vi "Data.vi"() -> ()   [LabVIEW 2015]
uses:
  <vilib>/addons/control/pid/pid.llb/PID (DBL).vi
  WINDOWS/system32/wlmData.dll
  <vilib>/addons/control/pid/NI_PID_pid.lvlib
panel:
  in  "output range CH4":cluster{"output high":dbl, "output low":dbl}={"output high"=2.5, "output low"=-2.5}
  in  "output range CH3":cluster{"output high":dbl, "output low":dbl}={"output high"=2.5, "output low"=-2.5}
  in  "output range CH2":cluster{"output high":dbl, "output low":dbl}={"output high"=2.5, "output low"=-2.5}
  in  "output range CH1":cluster{"output high":dbl, "output low":dbl}={"output high"=2.5, "output low"=-2.5}
  in  "Set p2":bool
  in  "Set f CH4 (THz) p2":dbl=811.289308 format="%.6f"
  in  "Set f CH3 (THz) p2":dbl=320.57268 format="%.6f"
  in  "Set f CH2 (THz) p2":dbl=751.527688 format="%.6f"
  in  "Set f CH1 (THz) p2":dbl=405.646266 format="%.6f"
  in  "Set p1":bool
  in  "Set f CH4 (THz) p1":dbl=811.289308 format="%.6f"
  in  "Set f CH3 (THz) p1":dbl=320.56993 format="%.6f"
  in  "Set f CH2 (THz) p1":dbl=751.52853 format="%.6f"
  in  "Set f CH1 (THz) p1":dbl=405.64502 format="%.6f"
  in  "Active interval CH4 (MHz)":dbl=100000.0
  in  "Zero CH4":bool
  in  "PID Out CH4(V)":dbl
  in  "PID gains CH4":T1={"proportional gain (Kc)"=1e-05, "integral time (Ti, min)"=0.0005, "derivative time (Td, min)"=0.0} {"derivative time (Td, min)" format="%.9f"; "integral time (Ti, min)" format="%.9f"; "proportional gain (Kc)" format="%.9f"}
  in  "Reinitialize PID CH4 (F)":bool
  in  "Inverse CH4":bool=TRUE
  out "df CH4 (MHz)":dbl format="%#.1f"
  out "Current f CH4 (THz)":dbl format="%#_9g"
  out "CH4 Reading":bool
  in  "Lock CH4":bool
  in  "Set f CH4 (THz)":dbl=811.289308 format="%.6f"
  out "df CH4 Chart (MHz)":dbl(graph)
  in  "PID Out CH3(V)":dbl
  in  "Zero CH3":bool
  in  "Active interval CH3 (MHz)":dbl=100000.0
  in  "PID gains CH3":T1={"proportional gain (Kc)"=1e-05, "integral time (Ti, min)"=0.0005, "derivative time (Td, min)"=0.0} {"derivative time (Td, min)" format="%.9f"; "integral time (Ti, min)" format="%.9f"; "proportional gain (Kc)" format="%.9f"}
  in  "Reinitialize PID CH3 (F)":bool
  in  "Inverse CH3":bool=TRUE
  out "df CH3 (MHz)":dbl=0.3482338115645689 format="%#.1f"
  out "Current f CH3 (THz)":dbl=320.5699303482334 format="%#_9g"
  out "CH3 Reading":bool
  in  "Lock CH3":bool
  in  "Set f CH3 (THz)":dbl=320.56993 format="%.6f"
  out "df CH3 Chart (MHz)":dbl(graph)=0.3482338115645689
  out "df CH2 Chart (MHz)":dbl(graph)=8543.924245259404
  in  "Zero CH2":bool
  in  "PID Out CH2(V)":dbl min=-10.0 max=10.0
  in  "Zero CH1":bool
  in  "PID Out CH1(V)":dbl
  out "df CH1 Chart (MHz)":dbl(graph)=-366.051154003344
  in  "PID gains CH2":T1={"proportional gain (Kc)"=1e-06, "integral time (Ti, min)"=1e-06, "derivative time (Td, min)"=0.0} {"derivative time (Td, min)" format="%.9f"; "integral time (Ti, min)" format="%.9f"; "proportional gain (Kc)" format="%.9f"}
  in  "Reinitialize PID CH2 (F)":bool
  in  "Inverse CH2":bool=TRUE
  out "df CH2 (MHz)":dbl=8543.924245259404 format="%#.1f"
  out "Current f CH2 (THz)":dbl=751.5362439242452 format="%#_9g"
  out "CH2 Reading":bool
  in  "Lock CH2":bool
  in  "Active interval CH2 (MHz) 2":dbl=100000.0
  in  "Set f CH2 (THz)":dbl=751.52853 format="%.6f"
  in  "Lock CH1":bool
  out "CH1 Reading":bool
  in  "Ch control":string="None"
  in  "Active interval CH1 (MHz)":dbl=100000.0
  out "Current f CH1 (THz)":dbl=405.644653948846 format="%#_9g"
  out "df CH1 (MHz)":dbl=-366.051154003344 format="%#.1f"
  in  "Inverse CH1":bool=TRUE
  in  "Reinitialize PID CH1 (F)":bool
  in  "Set f CH1 (THz)":dbl=405.64502 format="%.6f"
  in  "PID gains CH1":T1={"proportional gain (Kc)"=1e-05, "integral time (Ti, min)"=0.0005, "derivative time (Td, min)"=0.0} {"derivative time (Td, min)" format="%.9f"; "integral time (Ti, min)" format="%.9f"; "proportional gain (Kc)" format="%.9f"}
  out "Current f Reading (THz)":dbl=-3.0 format="%#_9g"
  # "399 nm"
  # "740 nm (370 nm)"
  # "935 nm"
  # "Preset 1 (YB 171)"
  # "Preset 2 (YB 174)"
  # "Physical port:\nDAQ1 AO0"
  # "Physical port:\nDAQ1 AO1"
  # "Physical port:\nDAQ2 AO0"
  # "Physical port:\nDAQ2 AO1"
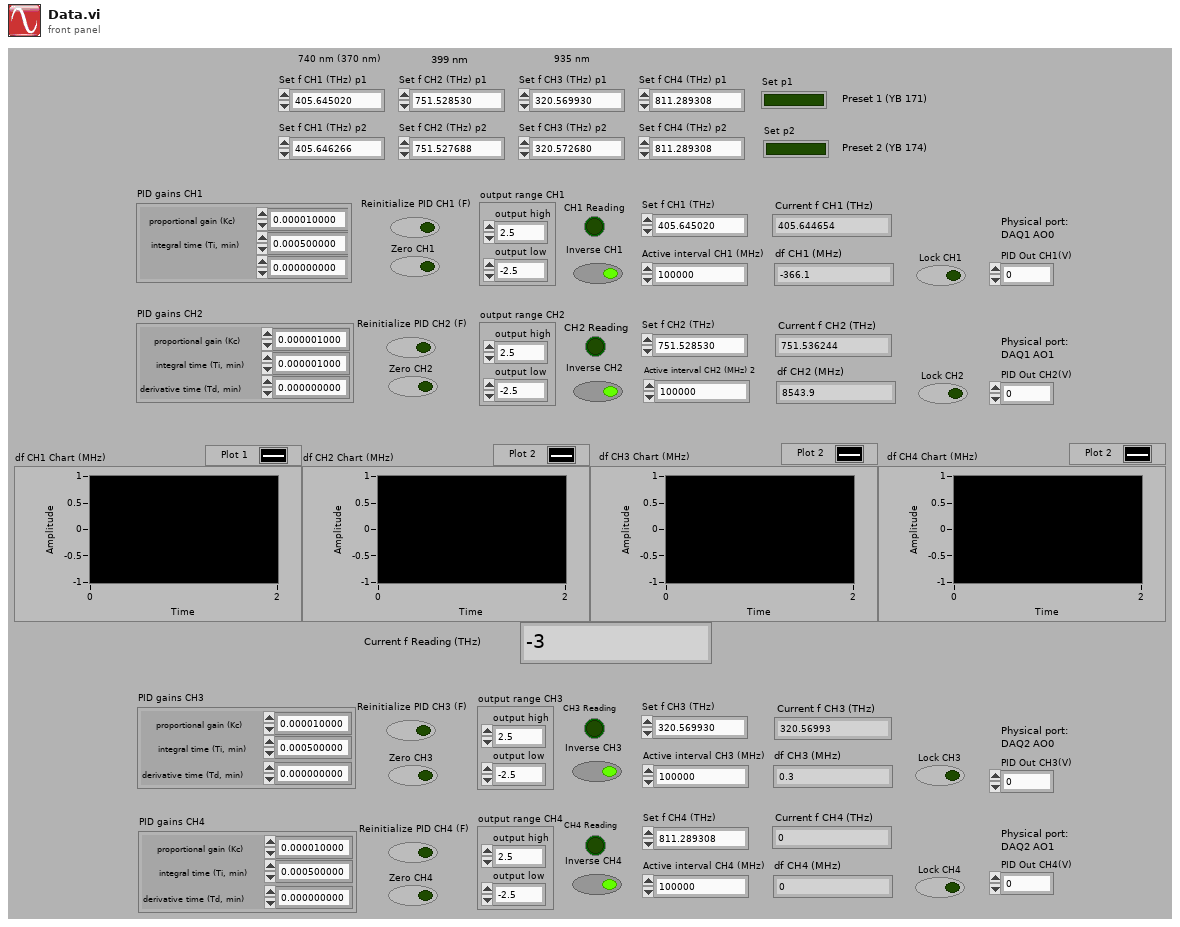
[diagram p1: front panel]
types:
  T1 = cluster{"proportional gain (Kc)":dbl, "integral time (Ti, min)":dbl, "derivative time (Td, min)":dbl}
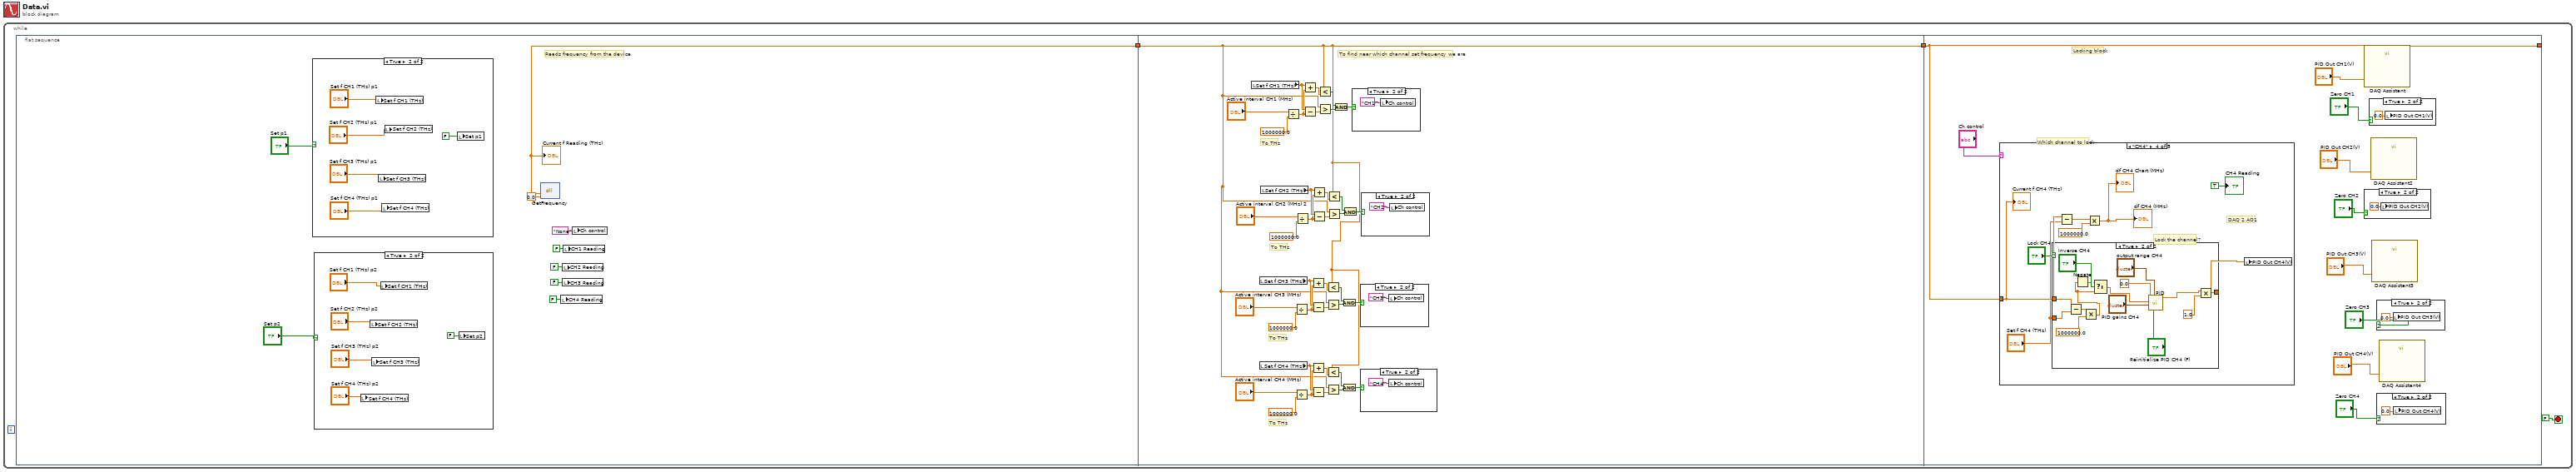
[diagram p0: block diagram]
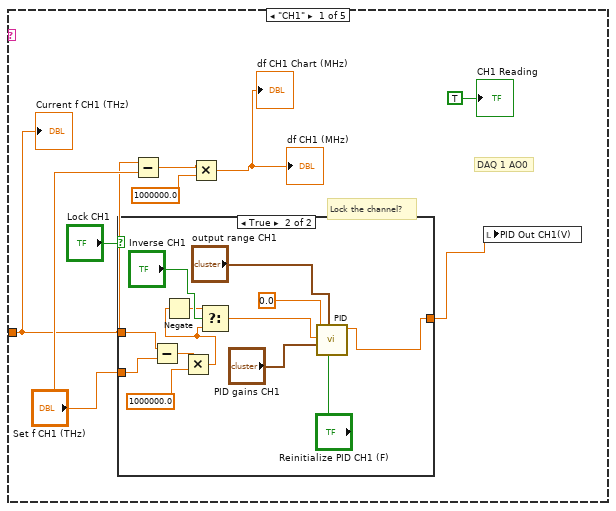
[diagram p12: hidden frame]
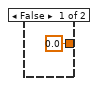
[diagram p13: hidden frame]
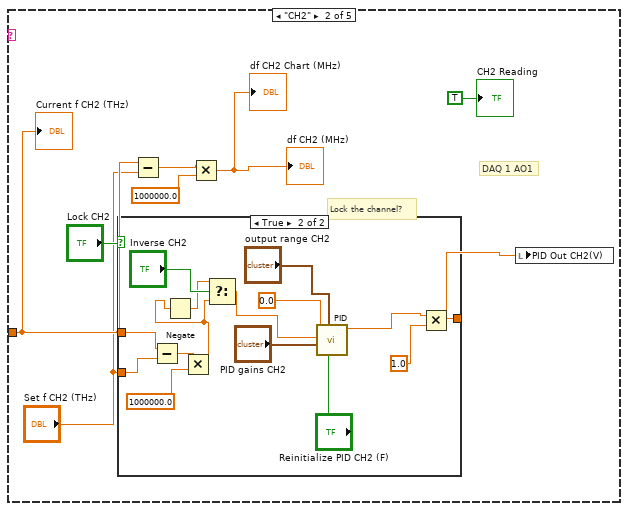
[diagram p14: hidden frame]
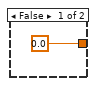
[diagram p15: hidden frame]
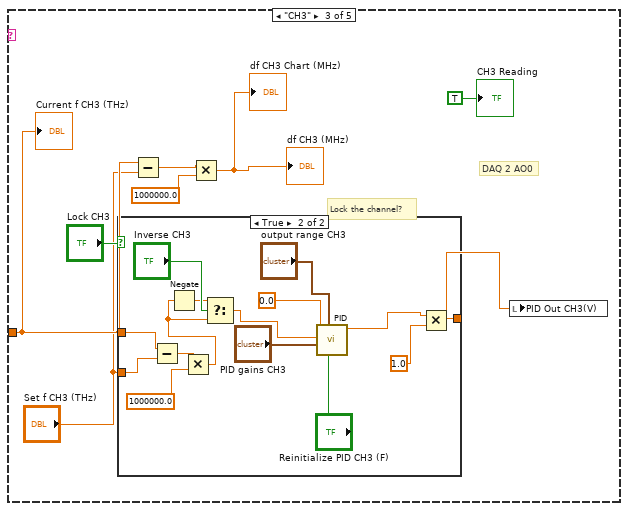
[diagram p16: hidden frame]
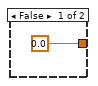
[diagram p17: hidden frame]
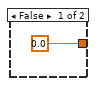
[diagram p18: hidden frame]
diagram:
  n1 = while {
    stop <- FALSE stop-if-true
    n2 = flat-sequence {
      tunnel: [w9] -> w2
      tunnel: w2 -> [w23]
      tunnel: [w23] -> w1
      tunnel: [w73] -> _
      tunnel: w1 -> [w73]
      frame #0 {
        # "Reads frequency from the device"
        n3 = case shown="True" "Set p1" {
          frame False {
          }
          frame True {
            n4 = local write "Set f CH1 (THz)"("Set f CH1 (THz) p1") -> ()
            n5 = local write "Set f CH3 (THz)"("Set f CH3 (THz) p1") -> ()
            n6 = local write "Set f CH4 (THz)"("Set f CH4 (THz) p1") -> ()
            n7 = local write "Set f CH2 (THz)"("Set f CH2 (THz) p1") -> ()
            n8 = local write "Set p1"(FALSE ("Set p1")) -> ()
          }
        }
        n9 = case shown="True" "Set p2" {
          frame False {
          }
          frame True {
            n10 = local write "Set f CH4 (THz)"("Set f CH4 (THz) p2") -> ()
            n11 = local write "Set f CH2 (THz)"("Set f CH2 (THz) p2") -> ()
            n12 = local write "Set f CH3 (THz)"("Set f CH3 (THz) p2") -> ()
            n13 = local write "Set f CH1 (THz)"("Set f CH1 (THz) p2") -> ()
            n14 = local write "Set p2"(FALSE ("Set p2")) -> ()
          }
        }
        n15 = dll-call lib="C:/WINDOWS/system32/wlmData.dll" fn="GetFrequency"("arg1"=0.0) -> ("return type"=w9:dbl)  [unwired: 4 in, 2 out]
        "Current f Reading (THz)" <- w9
        n16 = local write "CH4 Reading"(FALSE ("CH4 Reading")) -> ()
        n17 = local write "CH2 Reading"(FALSE ("CH2 Reading")) -> ()
        n18 = local write "CH3 Reading"(FALSE ("CH3 Reading")) -> ()
        n19 = local write "CH1 Reading"(FALSE ("CH1 reading")) -> ()
        n20 = local write "Ch control"("None" ("Ch control")) -> ()
      }
      frame #1 {
        # "To THz"
        # "To THz"
        # "To THz"
        # "To find near which channel set frequency we are"
        # "To THz"
        n21 = local read "Set f CH1 (THz)"() -> (w56:dbl)
        n22 = local read "Set f CH3 (THz)"() -> (w38:dbl)
        n23 = local read "Set f CH4 (THz)"() -> (w29:dbl)
        n24 = local read "Set f CH2 (THz)"() -> (w47:dbl)
        n25 = Divide(x="Active interval CH1 (MHz)", y=1000000.0) -> (x/y=w55:dbl)
        n26 = Divide(x="Active interval CH3 (MHz)", y=1000000.0) -> (x/y=w37:dbl)
        n27 = Divide(x="Active interval CH4 (MHz)", y=1000000.0) -> (x/y=w28:dbl)
        n28 = Divide(x="Active interval CH2 (MHz) 2", y=1000000.0) -> (x/y=w46:dbl)
        n29 = Add(x=w56, y=w55) -> (x+y=w57:dbl)
        n30 = Subtract(x=w56, y=w55) -> (x-y=w54:dbl)
        n31 = Add(x=w38, y=w37) -> (x+y=w39:dbl)
        n32 = Subtract(x=w38, y=w37) -> (x-y=w36:dbl)
        n33 = Add(x=w29, y=w28) -> (x+y=w30:dbl)
        n34 = Subtract(x=w29, y=w28) -> (x-y=w27:dbl)
        n35 = Add(x=w47, y=w46) -> (x+y=w48:dbl)
        n36 = Subtract(x=w47, y=w46) -> (x-y=w45:dbl)
        n37 = Less?(x=w23, y=w57) -> (x < y?=w53:bool)
        n38 = Greater?(x=w23, y=w54) -> (0:w52:bool)
        n39 = Less?(x=w23, y=w39) -> (x < y?=w35:bool)
        n40 = Greater?(x=w23, y=w36) -> (0:w34:bool)
        n41 = Less?(x=w23, y=w30) -> (x < y?=w26:bool)
        n42 = Greater?(x=w23, y=w27) -> (0:w25:bool)
        n43 = Less?(x=w23, y=w48) -> (x < y?=w44:bool)
        n44 = Greater?(x=w23, y=w45) -> (0:w43:bool)
        n45 = And(x=w53, y=w52) -> (x .and. y?=w51:bool)
        n46 = And(x=w35, y=w34) -> (x .and. y?=w33:bool)
        n47 = And(x=w26, y=w25) -> (x .and. y?=w24:bool)
        n48 = And(x=w44, y=w43) -> (x .and. y?=w42:bool)
        n49 = case shown="True" w51 {
          frame False {
          }
          frame True {
            n50 = local write "Ch control"("CH1" ("Ch control")) -> ()
          }
        }
        n51 = case shown="True" w33 {
          frame False {
          }
          frame True {
            n52 = local write "Ch control"("CH3" ("Ch control")) -> ()
          }
        }
        n53 = case shown="True" w24 {
          frame False {
          }
          frame True {
            n54 = local write "Ch control"("CH4" ("Ch control")) -> ()
          }
        }
        n55 = case shown="True" w42 {
          frame False {
          }
          frame True {
            n56 = local write "Ch control"("CH2" ("Ch control")) -> ()
          }
        }
      }
      frame #2 {
        # "Which channel to lock"
        # "Locking block"
        n57 = case shown="\"CH4\"" "Ch control" {
          tunnel: w73 -> [w84 w107 w131 w155 _]
          frame "CH1" {
            # "DAQ 1 AO0"
            # "Lock the channel?"
            n58 = case shown="True" "Lock CH1" {
              tunnel: "Set f CH1 (THz)" -> [_ w92]
              tunnel: w84 -> [_ w93]
              tunnel: [0.0 ("output") w89] -> w78
              frame False {
              }
              frame True {
                n59 = Subtract(x=w93, y=w92) -> (x-y=w91:dbl)
                n60 = Multiply(x=w91, y=1000000.0) -> (x*y=w87:dbl)
                n61 = Negate(x=w87) -> (-x=w95:dbl)
                n62 = Select(t=w95, s="Inverse CH1", f=w87) -> (s? t:f=w88:dbl)
                n63 = call-poly <vilib>:"PID.vi"("reinitialize? (F)"="Reinitialize PID CH1 (F)", "output range"="output range CH1", "PID gains"="PID gains CH1", "process variable"=w88, "setpoint"=0.0) -> ("output"=w89:dbl)  [unwired: 5 in, 1 out]
              }
            }
            n64 = Subtract(x=w84, y="Set f CH1 (THz)") -> (x-y=w82:dbl)
            n65 = Multiply(x=w82, y=1000000.0) -> (x*y=→"df CH1 (MHz)" →"df CH1 Chart (MHz)":dbl)
            n66 = local write "PID Out CH1(V)"(w78) -> ()
            "Current f CH1 (THz)" <- w84
            "CH1 Reading" <- TRUE ("CH1 reading")
          }
          frame "CH2" {
            # "DAQ 1 AO1"
            # "Lock the channel?"
            n67 = case shown="True" "Lock CH2" {
              tunnel: "Set f CH2 (THz)" -> [_ w116]
              tunnel: w107 -> [_ w117]
              tunnel: [0.0 ("output") w113] -> w101
              frame False {
              }
              frame True {
                n68 = Subtract(x=w117, y=w116) -> (x-y=w115:dbl)
                n69 = Multiply(x=w115, y=1000000.0) -> (x*y=w109:dbl)
                n70 = Negate(x=w109) -> (-x=w119:dbl)
                n71 = Select(t=w119, s="Inverse CH2", f=w109) -> (s? t:f=w110:dbl)
                n72 = call-poly <vilib>:"PID.vi"("reinitialize? (F)"="Reinitialize PID CH2 (F)", "output range"="output range CH2", "PID gains"="PID gains CH2", "process variable"=w110, "setpoint"=0.0) -> ("output"=w111:dbl)  [unwired: 5 in, 1 out]
                n73 = Multiply(x=w111, y=1.0) -> (x*y=w113:dbl)
              }
            }
            n74 = Subtract(x=w107, y="Set f CH2 (THz)") -> (x-y=w105:dbl)
            n75 = Multiply(x=w105, y=1000000.0) -> (x*y=→"df CH2 (MHz)" →"df CH2 Chart (MHz)":dbl)
            n76 = local write "PID Out CH2(V)"(w101) -> ()
            "Current f CH2 (THz)" <- w107
            "CH2 Reading" <- TRUE ("CH1 reading")
          }
          frame "CH3" {
            # "DAQ 2 AO0"
            # "Lock the channel?"
            n77 = case shown="True" "Lock CH3" {
              tunnel: "Set f CH3 (THz)" -> [_ w140]
              tunnel: w131 -> [_ w141]
              tunnel: [0.0 ("output") w137] -> w124
              frame False {
              }
              frame True {
                n78 = Subtract(x=w141, y=w140) -> (x-y=w139:dbl)
                n79 = Multiply(x=w139, y=1000000.0) -> (x*y=w133:dbl)
                n80 = Negate(x=w133) -> (-x=w143:dbl)
                n81 = Select(t=w143, s="Inverse CH3", f=w133) -> (s? t:f=w134:dbl)
                n82 = call-poly <vilib>:"PID.vi"("reinitialize? (F)"="Reinitialize PID CH3 (F)", "output range"="output range CH3", "PID gains"="PID gains CH3", "process variable"=w134, "setpoint"=0.0) -> ("output"=w135:dbl)  [unwired: 5 in, 1 out]
                n83 = Multiply(x=w135, y=1.0) -> (x*y=w137:dbl)
              }
            }
            n84 = Subtract(x=w131, y="Set f CH3 (THz)") -> (x-y=w129:dbl)
            n85 = Multiply(x=w129, y=1000000.0) -> (x*y=→"df CH3 (MHz)" →"df CH3 Chart (MHz)":dbl)
            n86 = local write "PID Out CH3(V)"(w124) -> ()
            "Current f CH3 (THz)" <- w131
            "CH3 Reading" <- TRUE ("CH1 reading")
          }
          frame "CH4" {
            # "DAQ 2 AO1"
            # "Lock the channel?"
            n87 = case shown="True" "Lock CH4" {
              tunnel: "Set f CH4 (THz)" -> [_ w164]
              tunnel: w155 -> [_ w165]
              tunnel: [0.0 ("output") w161] -> w149
              frame False {
              }
              frame True {
                n88 = Subtract(x=w165, y=w164) -> (x-y=w163:dbl)
                n89 = Multiply(x=w163, y=1000000.0) -> (x*y=w157:dbl)
                n90 = Negate(x=w157) -> (-x=w167:dbl)
                n91 = Select(t=w167, s="Inverse CH4", f=w157) -> (s? t:f=w158:dbl)
                n92 = call-poly <vilib>:"PID.vi"("reinitialize? (F)"="Reinitialize PID CH4 (F)", "output range"="output range CH4", "PID gains"="PID gains CH4", "process variable"=w158, "setpoint"=0.0) -> ("output"=w159:dbl)  [unwired: 5 in, 1 out]
                n93 = Multiply(x=w159, y=1.0) -> (x*y=w161:dbl)
              }
            }
            n94 = Subtract(x=w155, y="Set f CH4 (THz)") -> (x-y=w153:dbl)
            n95 = Multiply(x=w153, y=1000000.0) -> (x*y=→"df CH4 (MHz)" →"df CH4 Chart (MHz)":dbl)
            n96 = local write "PID Out CH4(V)"(w149) -> ()
            "Current f CH4 (THz)" <- w155
            "CH4 Reading" <- TRUE ("CH1 reading")
          }
          frame Default {
          }
        }
        n97 = call "DAQ Assistant"("data"="PID Out CH1(V)") -> ()  [unwired: 17 in, 2 out]
        n98 = case shown="True" "Zero CH2" {
          frame False {
          }
          frame True {
            n99 = local write "PID Out CH2(V)"(0.0 ("data")) -> ()
          }
        }
        n100 = case shown="True" "Zero CH1" {
          frame False {
          }
          frame True {
            n101 = local write "PID Out CH1(V)"(0.0 ("data")) -> ()
          }
        }
        n102 = call "DAQ Assistant2"("data"="PID Out CH2(V)") -> ()  [unwired: 17 in, 2 out]
        n103 = call "DAQ Assistant3"("data"="PID Out CH3(V)") -> ()  [unwired: 17 in, 2 out]
        n104 = case shown="True" "Zero CH3" {
          frame False {
          }
          frame True {
            n105 = local write "PID Out CH3(V)"(0.0 ("data")) -> ()
          }
        }
        n106 = case shown="True" "Zero CH4" {
          frame False {
          }
          frame True {
            n107 = local write "PID Out CH4(V)"(0.0 ("data")) -> ()
          }
        }
        n108 = call "DAQ Assistant4"("data"="PID Out CH4(V)") -> ()  [unwired: 17 in, 2 out]
      }
    }
  }
